vi "RGB to Gray.vi"(8 "error in (no error)":errorcluster caption="错误输入（无错误）", 11 "image data":T1 caption="图像数据") -> (0 "error out":errorcluster caption="错误输出", 3 "输出簇":T1)   [LabVIEW 2012, in "Picture Box Tools.lvlib"]
uses:
  <vilib>/picture/picture.llb/imagedata.ctl
  Picture Box Tools.lvlib
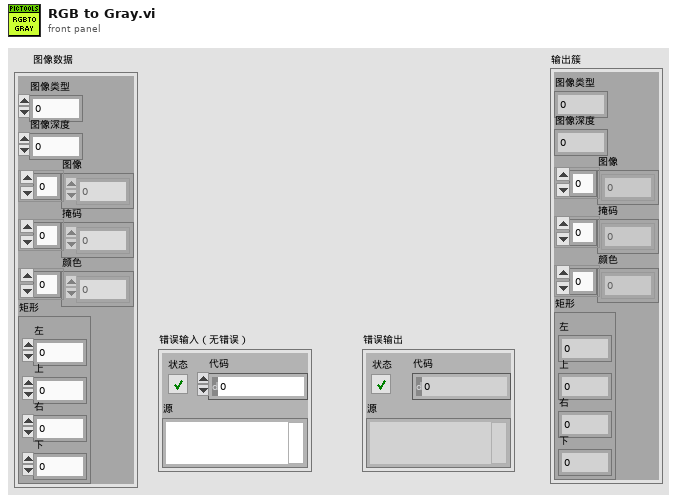
[diagram p1: front panel]
types:
  T1 = typedef "imagedata.ctl" = cluster{"image type":i32, "image depth":i32, "image":u8[], "mask":u8[], "colors":u32[], "Rectangle":cluster{"left":i16, "top":i16, "right":i16, "bottom":i16}}
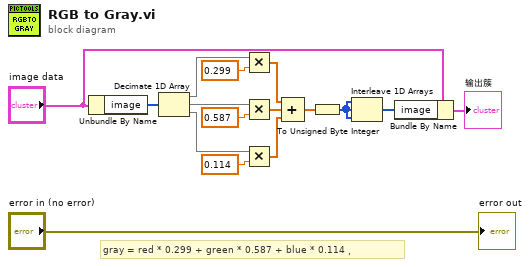
[diagram p0: block diagram]
diagram:
  # "gray = red * 0.299 + green * 0.587 + blue * 0.114，"
  n1 = Unbundle By Name("image data") -> ("image"=w16:u8[])
  n2 = Decimate 1D Array(w16) -> (w15:u8[], w13:u8[], w11:u8[])
  n3 = Multiply(x=w15, y=0.299) -> (x*y=w9:dbl[])
  n4 = Multiply(x=w13, y=0.587) -> (x*y=w8:dbl[])
  n5 = Multiply(x=w11, y=0.114) -> (x*y=w7:dbl[])
  n6 = Compound Arithmetic op=ADD(w9, w8, w7) -> (w6:dbl[])
  n7 = To Unsigned Byte Integer(number=w6) -> (unsigned 8bit integer=w2:u8[])
  n8 = Interleave 1D Arrays(w2, w2, w2) -> (w1:u8[])
  n9 = Bundle By Name(cluster="image data", "image"=w1) -> (→"输出簇":T1)
  "error out" <- "error in (no error)"
